vi "new report subVI.vi"(0 "report in":refnum<class "NI_Standard Report.lvclass">, 1 "window state (normal)":T1(ring)=enum."normal", 5 "display alerts? (F)":bool, 7 "template (empty)":path, 9 "machine name (empty)":string, 11 "error in (no error)":errorcluster) -> (4 "report out":refnum<class "NI_Standard Report.lvclass">, 15 "error out":errorcluster)   [LabVIEW 2017, in "NI_Standard Report.lvclass"]
uses:
  <vilib>/Utility/NIReport.llb/Standard Report/NI_Standard Report.lvclass
  <vilib>/Utility/NIReport.llb/Standard Report/NI_Standard Report.lvclass/NI_Standard Report.ctl
panel:
  in  "NIReports.Report":refnum<k7>
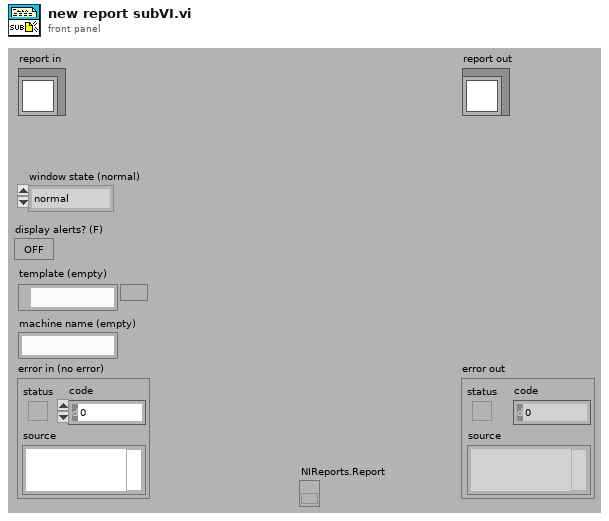
[diagram p1: front panel]
types:
  T1 = enum16{"maximized", "minimized", "normal", "no change"}
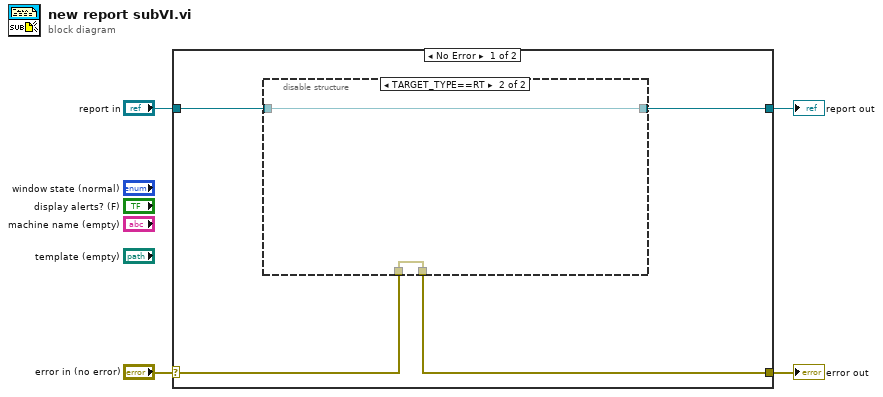
[diagram p0: block diagram]
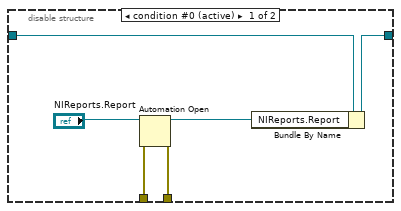
[diagram p2: hidden frame]
diagram:
  n1 = case shown="No Error" "error in (no error)" {
    selector: "error in (no error)" -> [w6 w18]
    tunnel: [w5 w18] -> w3
    tunnel: [w7 w17] -> w1
    tunnel: "report in" -> [w8 w17]
    frame No Error {
      n2 = disable-structure shown="TARGET_TYPE==RT" {
        disable-tunnel: w8 -> [w14 w16]
        disable-tunnel: [w13 w16] -> w7
        disable-tunnel: w6 -> [w10 w15]
        disable-tunnel: [w9 w15] -> w5
        frame condition #0 (active) {
          n3 = Automation Open(error in (no error)=w10, Automation Refnum="NIReports.Report") -> (Automation Refnum=w11:refnum<k7>, error out=w9:errorcluster)  [unwired: 2 out]
          n4 = Bundle By Name(cluster=w14, "NIReports.Report"=w11) -> (w13:refnum<class "NI_Standard Report.lvclass">)
        }
        frame condition #1 {
        }
      }
    }
    frame Error {
    }
  }
  "error out" <- w3
  "report out" <- w1
